vi "Serial Read-Write with timeout (VISA).vi"(4 "error in (no error)":errorcluster, 5 "Write String":string, 7 "VISA session":refnum<visa-resource-name>) -> (0 "error out":errorcluster, 1 "Speed":i16, 2 "status":u8[](array[numeric]), 3 "VISA session out":refnum<visa-resource-name>)   [LabVIEW 2019]
doc: "This vi is a simple and fast way to perform serial communication with other devices.\nIt uses Labview standard routines (do not use VISA).\nA time out of fail (1 second) is set if no answer is read on to input buffer."
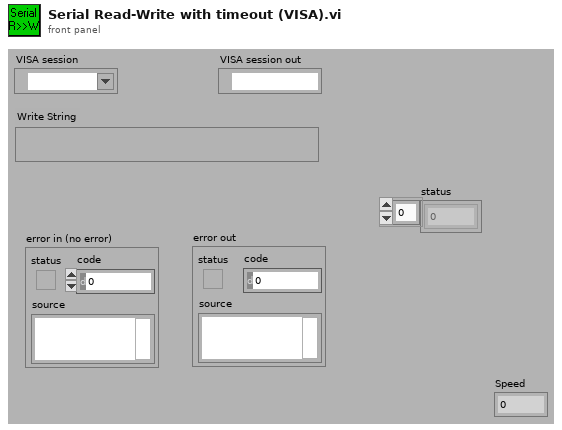
[diagram p1: front panel]
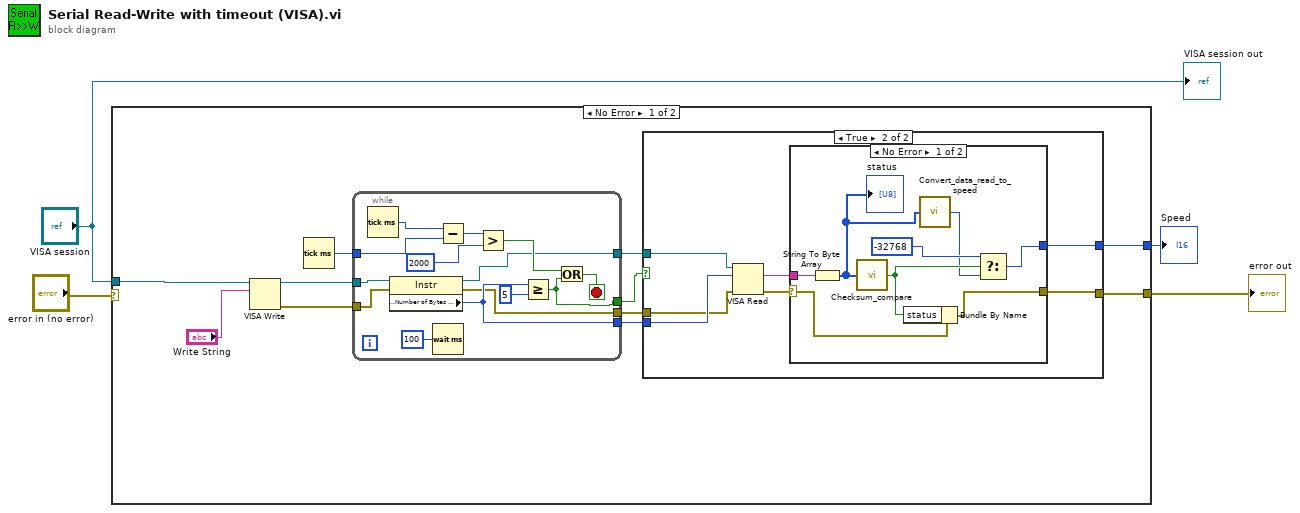
[diagram p0: block diagram]
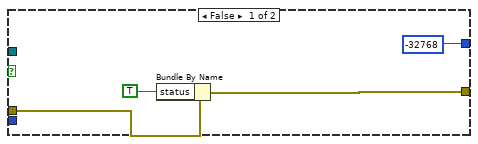
[diagram p2: hidden frame]
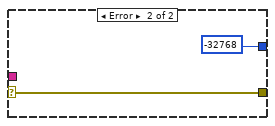
[diagram p3: hidden frame]
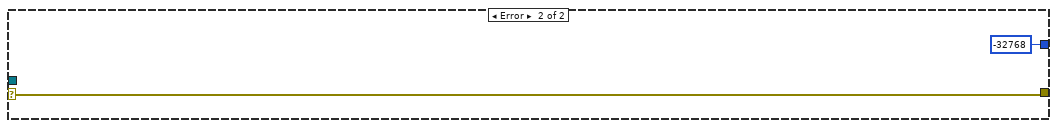
[diagram p4: hidden frame]
diagram:
  n1 = case shown="No Error" "error in (no error)" {
    selector: "error in (no error)" -> [_ w52]
    tunnel: [w8 w52] -> w3
    tunnel: "VISA session" -> [w6 _]
    tunnel: [w5 i16 -32768 ("Speed")] -> w1
    frame No Error {
      n2 = VISA Write(VISA resource name=w6, write buffer="Write String") -> (VISA resource name out=w13:refnum<visa-resource-name>, error out=w10:errorcluster)  [unwired: 1 in, 1 out]
      n3 = Tick Count (ms)() -> (millisecond timer value=w14:u32)
      n4 = while {
        tunnel: w14 -> [w45]
        tunnel: w13 -> [w42]
        tunnel: [w41] -> w12
        tunnel: [w40] -> w11
        tunnel: w10 -> [w39]
        tunnel: [w38] -> w9
        tunnel: [w37] -> w7
        stop <- w48 stop-if-true
        n5 = Tick Count (ms)() -> (millisecond timer value=w44:u32)
        n6 = property class="Instr"(reference=w42, error in=w39) -> (reference out=w41:refnum<visa-resource-name>, error out=w38:errorcluster, "Serial Settings:Number of Bytes at Serial Port"=w40:u32)
        n7 = Wait (ms)(milliseconds to wait=u32 100) -> ()  [unwired: 1 out]
        n8 = Subtract(x=w44, y=w45) -> (x-y=w50:u32)
        n9 = Greater?(x=w50, y=u32 2000) -> (0:w47:bool)
        n10 = Greater Or Equal?(x=w40, y=u32 5) -> (x >= y?=w37:bool)
        n11 = Or(x=w47, y=w37) -> (x .or. y?=w48:bool)
      }
      n12 = case shown="True" w7 {
        tunnel: w12 -> [_ w26]
        tunnel: w11 -> [_ w25]
        tunnel: w9 -> [w19 w24]
        tunnel: [w18 w21] -> w8
        tunnel: [i16 -32768 ("Speed") w20] -> w5
        frame False {
          n13 = Bundle By Name(cluster=w19, "status"=TRUE) -> (w18:errorcluster)
        }
        frame True {
          n14 = VISA Read(VISA resource name=w26, byte count=w25, error in (no error)=w24) -> (read buffer=w22:string, error out=w23:errorcluster)  [unwired: 2 out]
          n15 = case shown="No Error" w23 {
            selector: w23 -> [w32 w36]
            tunnel: w22 -> [w34 _]
            tunnel: [w33 w36] -> w21
            tunnel: [w29 i16 -32768 ("Speed")] -> w20
            frame No Error {
              n16 = String To Byte Array(string=w34) -> (unsigned byte array=w28:u8[])
              "status" <- w28
              n17 = call "Checksum_compare.vi"("Byte Array"=w28) -> ("Checksum <>?"=w31:bool)
              n18 = Bundle By Name(cluster=w32, "status"=w31) -> (w33:errorcluster)
              n19 = call "Convert_data_read_to_speed.vi"("Byte Array"=w28) -> ("Speed"=w27:i16)
              n20 = Select(t=i16 -32768 ("Speed"), s=w31, f=w27) -> (s? t:f=w29:i16)
            }
            frame Error {
            }
          }
        }
      }
    }
    frame Error {
    }
  }
  "error out" <- w3
  "Speed" <- w1
  "VISA session out" <- "VISA session"
